vi "pp3b_log_DAQconfig.vi"(10 "queue in":refnum<queue>, 11 "Daq config":T1={"Sound AO"="Dev6/ao0", "Shock intesity AO"="Dev6/ao1", "Code_LED DO"="Dev6/port1:2", "Switch DI"="Dev6/port1/line0", "Webcam"="cam9", "Sound AO task"="", "Sound card task"=0, "Shock intensity AO task"="", "Code_LED DO task"="", "Switch DI task"="", "AO <=> Sound card"=FALSE, "Sound card"=0, "sample rate"=100000.0, "Variable shock"=TRUE, "Webcam on"=FALSE, "Waveform memo"={"t0"=timestamp(0 s since 1904-01-01), "dt"=1.0, "Y"=[]}, "Tone trigger"="PFI1", "Master-9 DO"="", "Master-9 DO task"="Dev6/port0/line5:7", "Master-9 on"=TRUE} {"sample rate" min=8000.0; "Sound card task" format="%.0x"}) -> (2 "queue out":refnum<queue>)   [LabVIEW 2013]
uses:
  CTL_pp3c_DaqStatus.ctl
  <vilib>/userdefined/High Color/IMAQdx.ctl
  <vilib>/sound2/lvsound2.llb/Sound Output Task ID.ctl
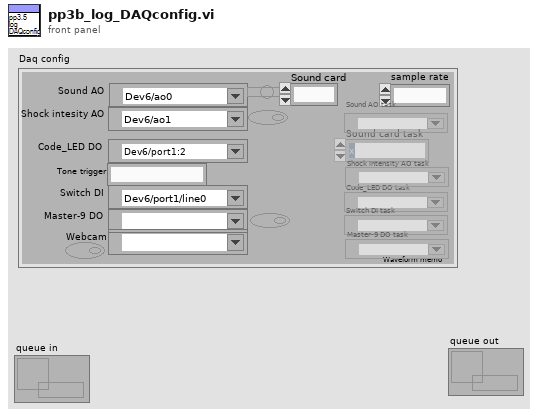
[diagram p1: front panel]
types:
  T1 = typedef "CTL_pp3c_DaqStatus.ctl" = cluster{"Sound AO":tag, "Shock intesity AO":tag, "Code_LED DO":tag, "Switch DI":tag, "Webcam":T2, "Sound AO task":refnum<k21>, "Sound card task":T3, "Shock intensity AO task":refnum<k21>, "Code_LED DO task":refnum<k21>, "Switch DI task":refnum<k21>, "AO <=> Sound card":bool, "Sound card":u32, "sample rate":dbl, "Variable shock":bool, "Webcam on":bool, "Waveform memo":waveform(dbl), "Tone trigger":string, "Master-9 DO":tag, "Master-9 DO task":refnum<k21>, "Master-9 on":bool}
  T2 = typedef "IMAQdx.ctl" = refnum<k21>
  T3 = typedef "Sound Output Task ID.ctl" = u32
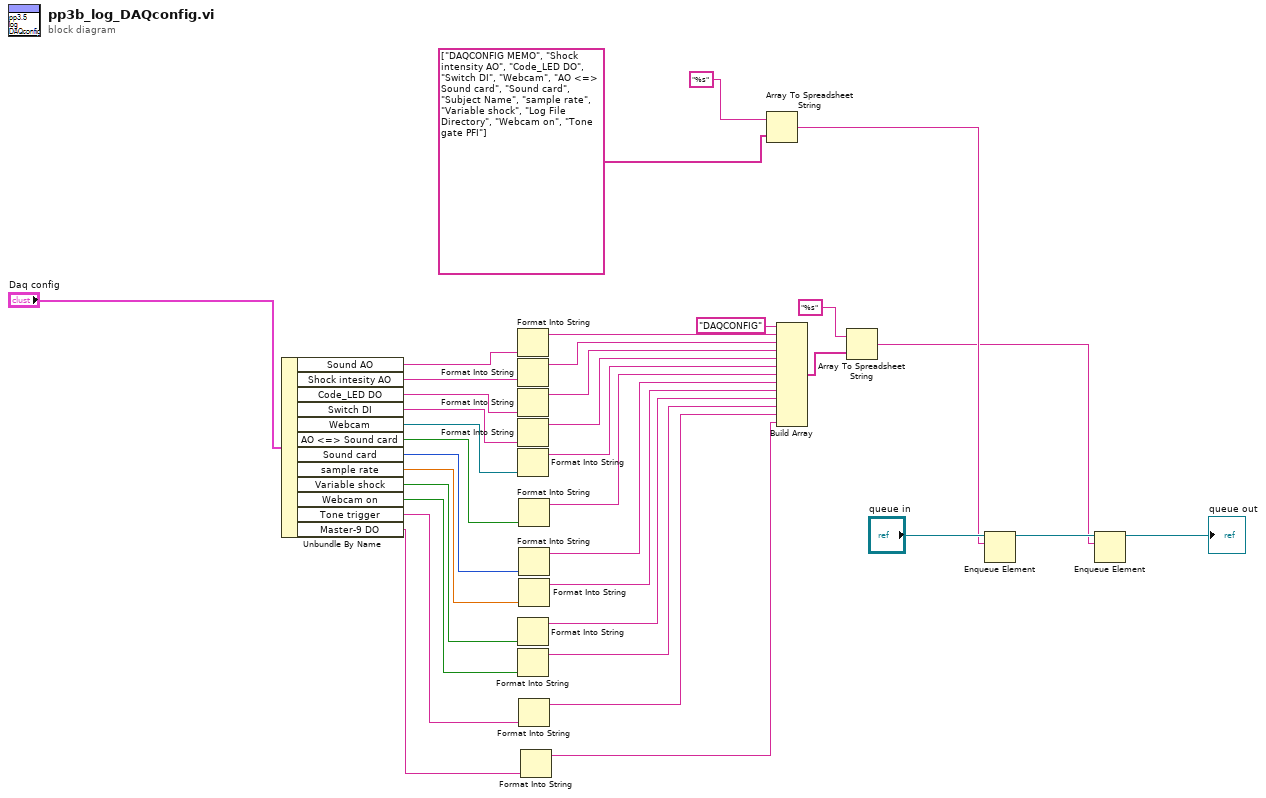
[diagram p0: block diagram]
diagram:
  n1 = Unbundle By Name("Daq config") -> ("Sound AO"=w35:tag, "Shock intesity AO"=w31:tag, "Code_LED DO"=w30:tag, "Switch DI"=w29:tag, "Webcam"=w28:T2, "AO <=> Sound card"=w27:bool, "Sound card"=w21:u32, "sample rate"=w20:dbl, "Variable shock"=w19:bool, "Webcam on"=w18:bool, "Tone trigger"=w17:string, "Master-9 DO"=w2:tag)
  n2 = Format Into String(w35) -> (resulting string=w33:string)  [unwired: 3 in, 1 out]
  n3 = Format Into String(w31) -> (resulting string=w26:string)  [unwired: 3 in, 1 out]
  n4 = Format Into String(w30) -> (resulting string=w25:string)  [unwired: 3 in, 1 out]
  n5 = Format Into String(w29) -> (resulting string=w24:string)  [unwired: 3 in, 1 out]
  n6 = Format Into String(w28) -> (resulting string=w23:string)  [unwired: 3 in, 1 out]
  n7 = Format Into String(w19) -> (resulting string=w14:string)  [unwired: 3 in, 1 out]
  n8 = Format Into String(w18) -> (resulting string=w13:string)  [unwired: 3 in, 1 out]
  n9 = Format Into String(w27) -> (resulting string=w22:string)  [unwired: 3 in, 1 out]
  n10 = Format Into String(w21) -> (resulting string=w16:string)  [unwired: 3 in, 1 out]
  n11 = Format Into String(w20) -> (resulting string=w15:string)  [unwired: 3 in, 1 out]
  n12 = Format Into String(w17) -> (resulting string=w12:string)  [unwired: 3 in, 1 out]
  n13 = Format Into String(w2) -> (resulting string=w1:string)  [unwired: 3 in, 1 out]
  n14 = Array To Spreadsheet String(array=string[] ["DAQCONFIG MEMO", "Shock intensity AO", "Code_LED DO", "Switch DI", "Webcam", "AO <=> Sound card", "Sound card", "Subject Name", "sample rate", "Variable shock", "Log File Directory", "Webcam on", "Tone gate PFI"], 3:"%s" ("format string")) -> (spreadsheet string=w4:string)  [unwired: 1 in]
  n15 = Build Array("DAQCONFIG" ("element"), w33, w26, w25, w24, w23, w22, w16, w15, w14, w13, w12, w1) -> (w10:string[])
  n16 = Array To Spreadsheet String(array=w10, 3:"%s" ("format string")) -> (spreadsheet string=w3:string)  [unwired: 1 in]
  n17 = Enqueue Element(queue="queue in", element=w4) -> (queue out=w6:refnum<queue>)  [unwired: 2 in, 2 out]
  n18 = Enqueue Element(queue=w6, element=w3) -> (queue out=→"queue out":refnum<queue>)  [unwired: 2 in, 2 out]
